vi "Temperature Limit.vi"(3 "상위 리미트":dbl=80.0 format="%.2f", 4 "델터 t(ms)":u32=400 min=50 max=2000 step=50, 5 "수집할 포인트":i32=75 min=20 max=500) -> ()   [LabVIEW 2010]
doc: "이 VI는 온도 수집을 시뮬레이션하며, 온도를 그래프로 나타내며, 온도가 리미트보다 높은 경우, 사용자에게 이를 통지합니다.\n\n이 VI는 LabVIEW Basics II의 연습문제이며 프로퍼티 노드를 배우는데 사용됩니다."
panel:
  out "리미트 초과":bool
  in  "강제 종료":bool
  out "온도":cluster{"Temperature":dbl, "High Limit":dbl}(graph)
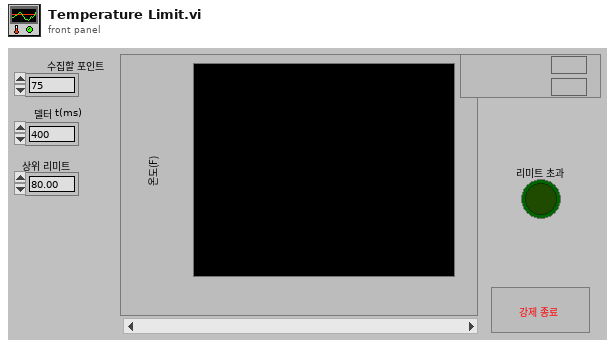
[diagram p1: front panel]
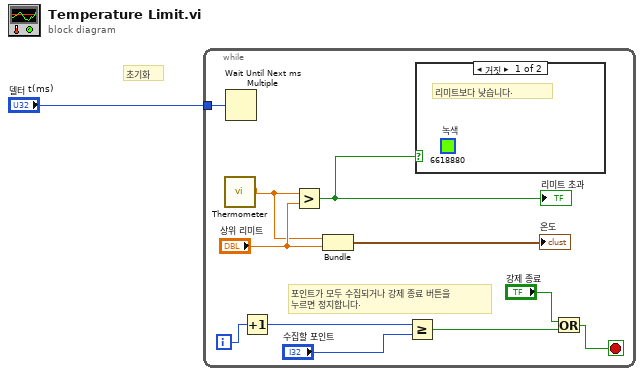
[diagram p0: block diagram]
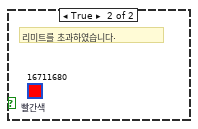
[diagram p2: hidden frame]
diagram:
  # "초기화"
  n1 = while {
    tunnel: "델터 t(ms)" -> [w4]
    i -> [w11]
    stop <- w5 stop-if-true
    # "포인트가 모두 수집되거나 강제 종료 버튼을 누르면 정지합니다."
    n2 = call "Thermometer.vi"() -> ("온도"=w2:dbl)  [unwired: 10 in, 1 out]
    n3 = Wait Until Next ms Multiple(millisecond multiple=w4) -> ()  [unwired: 1 out]
    n4 = Increment(x=w11) -> (x+1=w9:i32)
    n5 = Greater?(x=w2, y="상위 리미트") -> (0:w3:bool)
    "리미트 초과" <- w3
    n6 = Bundle("온도"=w2, "상위 리미트"="상위 리미트") -> (→"온도":cluster{"온도":dbl, "상위 리미트":dbl})  [unwired: 1 in]
    n7 = Greater Or Equal?(x=w9, y="수집할 포인트") -> (x >= y?=w7:bool)
    n8 = case shown="거짓" w3 {
      frame False {
        (unwired) u32 6618880  # 녹색
        # "리미트보다 낮습니다."
      }
      frame True {
        (unwired) u32 16711680  # 빨간색
        # "리미트를 초과하였습니다."
      }
    }
    n9 = Or(x="강제 종료", y=w7) -> (x .or. y?=w5:bool)
  }
